vi "Set Macro Active.vi"(8 "error in (no error)":errorcluster, 10 "Macro Name":string, 11 "Motions in":refnum<class "Motions.lvclass">) -> (0 "error out":errorcluster, 3 "Motions out":refnum<class "Motions.lvclass">)   [LabVIEW 2016, in "Hardware.lvlib" / "Motions.lvlib" / "Motions.lvclass"]
uses:
  <userlib>/Common Components/Hardware/Abstract System/Motions/Motions/Motions.lvclass
  <userlib>/Common Components/Hardware/Abstract System/Motions/Motions/Motions.lvclass/Motions.ctl
  <userlib>/Common Components/TriggerAction Q/TriggerAction Q/TriggerAction Q.lvclass
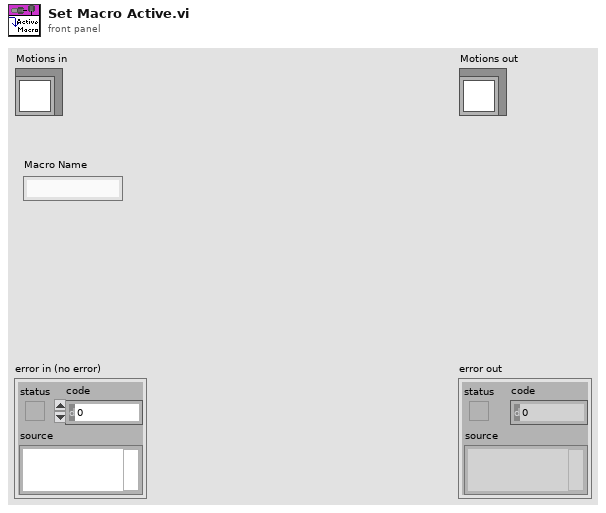
[diagram p1: front panel]
types:
  T1 = typedef "TriggerAction Q.lvclass/Element Data.ctl" = cluster{"Triggers":cluster{"Triggers for Array AND":string[]}[], "Actions":cluster{"Action Name":string, "Action Data":string}[]}
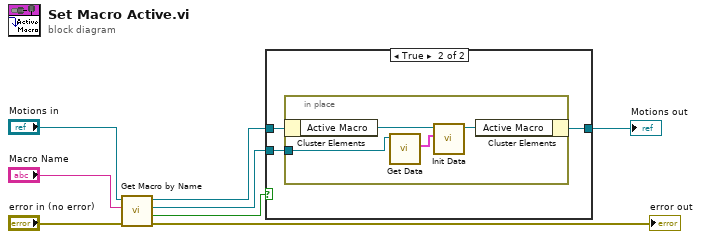
[diagram p0: block diagram]
diagram:
  n1 = call <userlib>:"Get Macro by Name.vi"("error in (no error)"="error in (no error)", "Macro Name"="Macro Name", "Motions in"="Motions in") -> ("error out"=→"error out":errorcluster, "found"=w4:bool, "TriggerAction Q.lvclass"=w2:refnum<class "TriggerAction Q.lvclass">, "Motions out"=w3:refnum<class "Motions.lvclass">)  [unwired: 5 in]
  n2 = case shown="True" w4 {
    tunnel: w3 -> [w9 w12]
    tunnel: w2 -> [_ w11]
    tunnel: [w9 w10] -> w1
    frame False {
    }
    frame True {
      n3 = in-place {
        in-place-border: w11 -> [w16]
        n4 = in-place-cluster #1(w12) -> ("Active Macro"=w15:refnum<class "TriggerAction Q.lvclass">)
        n5 = call <userlib>:"Get Data.vi"("TriggerAction in"=w16) -> ("Array of TriggerAction Elements"=w14:T1[])  [unwired: 8 in, 2 out]
        n6 = call <userlib>:"Init Data.vi"("Array of TriggerAction Elements"=w14, "TriggerAction in"=w15) -> ("TriggerAction out"=w13:refnum<class "TriggerAction Q.lvclass">)  [unwired: 8 in, 1 out]
        n7 = in-place-cluster #1("Active Macro"=w13) -> (w10:refnum<class "Motions.lvclass">)
      }
    }
  }
  "Motions out" <- w1
